vi "rqcBob Create.vi"(0 "FPGA resource":T1, 9 "bitfile version":string, 11 "error in":errorcluster) -> (4 "rqcBob out":refnum<class "rqcBob.lvclass">, 15 "error out":errorcluster)   [LabVIEW 2018, in "rqcBob.lvclass"]
uses:
  rqcBob.lvclass
  <vilib>/userdefined/Silver/nirio_resource_slv.ctl
  rqcBob.lvclass/rqcBob.ctl
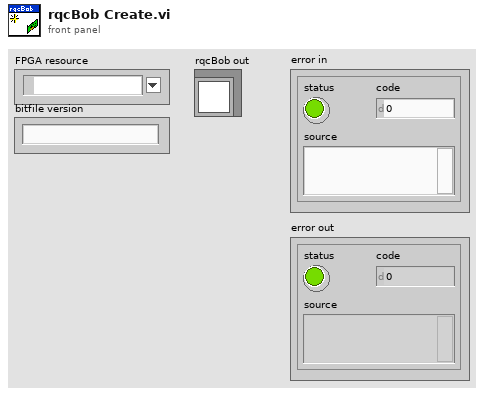
[diagram p1: front panel]
types:
  T1 = typedef "nirio_resource_slv.ctl" = tag
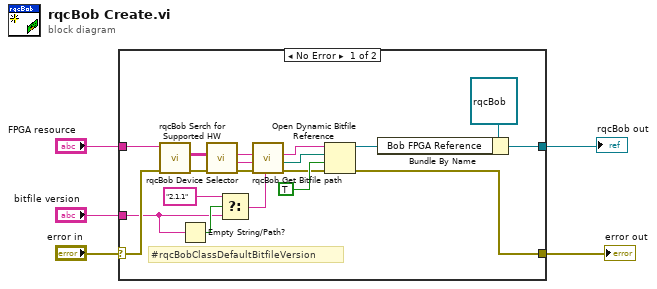
[diagram p0: block diagram]
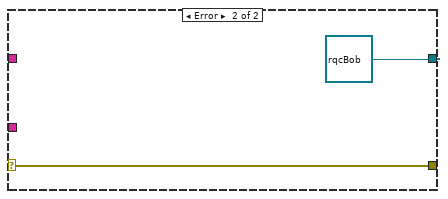
[diagram p2: hidden frame]
diagram:
  n1 = case shown="No Error" "error in" {
    selector: "error in" -> [w23 w26]
    tunnel: [w8 w26] -> w4
    tunnel: [w7 refnum<class "rqcBob.lvclass"> refnum ("rqcBob.lvclass")] -> w3
    tunnel: "FPGA resource" -> [w24 _]
    tunnel: "bitfile version" -> [w15 _]
    frame No Error {
      # "#rqcBobClassDefaultBitfileVersion"
      n2 = call "rqcBob Serch for Supported HW.vi"("error in"=w23, "Expected Resource Name"=w24) -> ("error out"=w22:errorcluster, "Compatible Devices List"=w21:string[][])  [unwired: 8 in]
      n3 = Empty String/Path?(string/path=w15) -> (empty?=w18:bool)
      n4 = call "rqcBob Device Selector.vi"("error in"=w22, "Compatible Devices List"=w21) -> ("error out"=w20:errorcluster, "Device"=w19:string, "Resource Name"=w12:string)  [unwired: 7 in]
      n5 = Select(t="2.1.1", s=w18, f=w15) -> (s? t:f=w16:string)
      n6 = call "rqcBob Get Bitfile path.vi"("bitfile version"=w16, "error in"=w20, "Device"=w19, "Resource Name"=w12) -> ("error out"=w13:errorcluster, "rqcBob Bitfile path"=w10:path, "Resource Name out"=w11:string)  [unwired: 4 in, 1 out]
      n7 = Open Dynamic Bitfile Reference(0:w11, 1:w10, 2:TRUE ("Run When Loaded"), 3:w13) -> (5:w9:refnum<k20>, 8:w8:errorcluster)  [unwired: 1 in]
      n8 = Bundle By Name(cluster=refnum<class "rqcBob.lvclass"> refnum ("rqcBob.lvclass"), "Bob FPGA Reference"=w9) -> (w7:refnum<class "rqcBob.lvclass">)
    }
    frame Error {
    }
  }
  "error out" <- w4
  "rqcBob out" <- w3
